vi "Abort.vi"(8 "error in (no error)":errorcluster, 11 "ChromaAcLoad in":refnum<class "ChromaAcLoad.lvclass">) -> (0 "error out":errorcluster, 3 "ChromaAcLoad out":refnum<class "ChromaAcLoad.lvclass">)   [LabVIEW 2018, in "AcPwrPlugins.lvlib" / "ChromaAcLoad.lvclass"]
uses:
  ChromaAcLoad.lvclass
  AcPwrBaseClass/AcPwrBase.lvclass
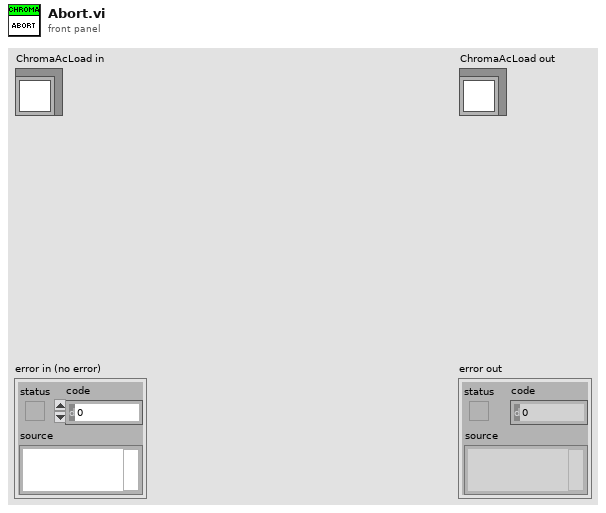
[diagram p1: front panel]
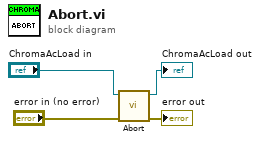
[diagram p0: block diagram]
diagram:
  n1 = call-parent "Abort.vi"("error in (no error)"="error in (no error)", "AcPwrBase in"="ChromaAcLoad in") -> ("error out"=→"error out":errorcluster, "AcPwrBase out"=→"ChromaAcLoad out":refnum<class "ChromaAcLoad.lvclass">)  [unwired: 8 in]
